vi "Apply.vi"(8 "Error In":errorcluster, 11 "object in":refnum<class "DS1054 Base CFG.lvclass">) -> (0 "Error Out":errorcluster, 3 "object out":refnum<class "DS1054 Base CFG.lvclass">)   [LabVIEW 2023, in "RIGOL DS1054Z.lvlib" / "DS1054 Base CFG.lvclass"]
uses:
  DS1054 Base CFG.lvclass
  DS1054 Base CFG.lvclass/DS1054 Base CFG.ctl
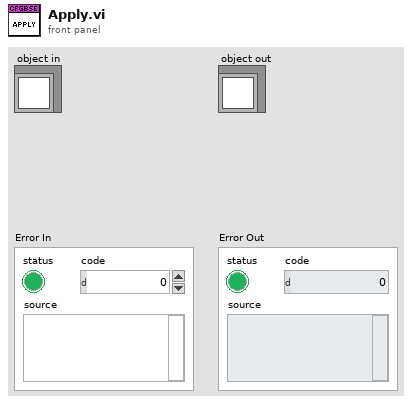
[diagram p1: front panel]
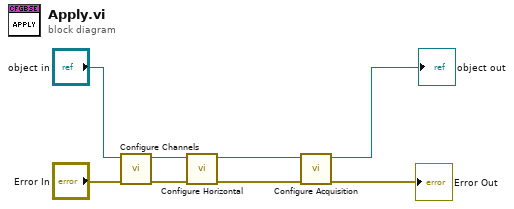
[diagram p0: block diagram]
diagram:
  n1 = call-dynamic "Configure Channels.vi"("error in"="Error In", "object in"="object in") -> ("error out"=w7:errorcluster, "object out"=w4:refnum<class "DS1054 Base CFG.lvclass">)  [unwired: 8 in]
  n2 = call-dynamic "Configure Horizontal.vi"("error in"=w7, "DS1054 Base CFG in"=w4) -> ("error out"=w5:errorcluster, "DS1054 Base CFG out"=w2:refnum<class "DS1054 Base CFG.lvclass">)  [unwired: 8 in]
  n3 = call-dynamic "Configure Acquisition.vi"("error in"=w5, "DS1054 Base CFG in"=w2) -> ("error out"=→"Error Out":errorcluster, "DS1054 Base CFG out"=→"object out":refnum<class "DS1054 Base CFG.lvclass">)  [unwired: 8 in]
